vi "DOselector.vi"(8 "I/O element":T1(ring), 11 "value":bool) -> ()   [LabVIEW 2024]
uses:
  <vilib>/eio/EIONode/EIONode.xnode
  <vilib>/rvi/eio/common/nirviEmuTemplateMethod_errors.vi
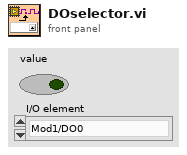
[diagram p1: front panel]
types:
  T1 = enum16{"Mod1/DO0", "Mod1/DO1", "Mod1/DO2", "Mod1/DO3", "Mod1/DO4", "Mod1/DO5", "Mod1/DO6", "Mod1/DO7", "Mod2/DIO0", "Mod2/DIO1", "Mod2/DIO2", "Mod2/DIO3", "Mod2/DIO4", "Mod2/DIO5", "Mod2/DIO6", "Mod2/DIO7"}
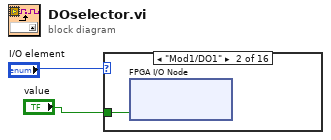
[diagram p0: block diagram]
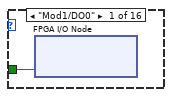
[diagram p2: hidden frame]
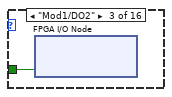
[diagram p3: hidden frame]
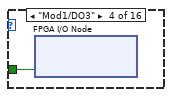
[diagram p4: hidden frame]
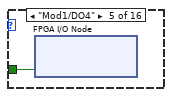
[diagram p5: hidden frame]
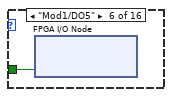
[diagram p6: hidden frame]
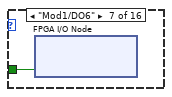
[diagram p7: hidden frame]
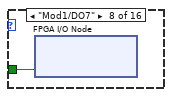
[diagram p8: hidden frame]
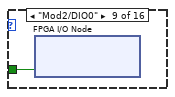
[diagram p9: hidden frame]
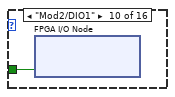
[diagram p10: hidden frame]
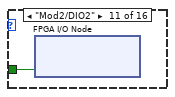
[diagram p11: hidden frame]
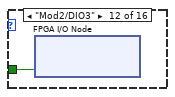
[diagram p12: hidden frame]
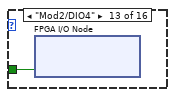
[diagram p13: hidden frame]
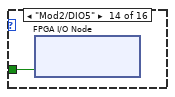
[diagram p14: hidden frame]
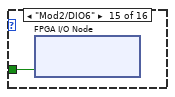
[diagram p15: hidden frame]
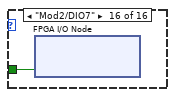
[diagram p16: hidden frame]
diagram:
  n1 = case shown="\"Mod1/DO1\"" "I/O element" {
    tunnel: "value" -> [w3 w4 w5 w6 w7 w8 w9 w10 w11 w12 w13 w14 w15 w16 w17 w18]
    frame "Mod1/DO0" {
      n2 = xnode "FPGA I/O Node"("Mod1/DO0"=w3) -> ()  [unwired: 2 in, 2 out]
    }
    frame "Mod1/DO1" {
      n3 = xnode "FPGA I/O Node"("Mod1/DO1"=w4) -> ()  [unwired: 2 in, 2 out]
    }
    frame "Mod1/DO2" {
      n4 = xnode "FPGA I/O Node"("Mod1/DO2"=w5) -> ()  [unwired: 2 in, 2 out]
    }
    frame "Mod1/DO3" {
      n5 = xnode "FPGA I/O Node"("Mod1/DO3"=w6) -> ()  [unwired: 2 in, 2 out]
    }
    frame "Mod1/DO4" {
      n6 = xnode "FPGA I/O Node"("Mod1/DO4"=w7) -> ()  [unwired: 2 in, 2 out]
    }
    frame "Mod1/DO5" {
      n7 = xnode "FPGA I/O Node"("Mod1/DO5"=w8) -> ()  [unwired: 2 in, 2 out]
    }
    frame "Mod1/DO6" {
      n8 = xnode "FPGA I/O Node"("Mod1/DO6"=w9) -> ()  [unwired: 2 in, 2 out]
    }
    frame "Mod1/DO7" {
      n9 = xnode "FPGA I/O Node"("Mod1/DO7"=w10) -> ()  [unwired: 2 in, 2 out]
    }
    frame "Mod2/DIO0" {
      n10 = xnode "FPGA I/O Node"("Mod2/DIO0"=w11) -> ()  [unwired: 2 in, 2 out]
    }
    frame "Mod2/DIO1" {
      n11 = xnode "FPGA I/O Node"("Mod2/DIO1"=w12) -> ()  [unwired: 2 in, 2 out]
    }
    frame "Mod2/DIO2" {
      n12 = xnode "FPGA I/O Node"("Mod2/DIO2"=w13) -> ()  [unwired: 2 in, 2 out]
    }
    frame "Mod2/DIO3" {
      n13 = xnode "FPGA I/O Node"("Mod2/DIO3"=w14) -> ()  [unwired: 2 in, 2 out]
    }
    frame "Mod2/DIO4" {
      n14 = xnode "FPGA I/O Node"("Mod2/DIO4"=w15) -> ()  [unwired: 2 in, 2 out]
    }
    frame "Mod2/DIO5" {
      n15 = xnode "FPGA I/O Node"("Mod2/DIO5"=w16) -> ()  [unwired: 2 in, 2 out]
    }
    frame "Mod2/DIO6" {
      n16 = xnode "FPGA I/O Node"("Mod2/DIO6"=w17) -> ()  [unwired: 2 in, 2 out]
    }
    frame "Mod2/DIO7" {
      n17 = xnode "FPGA I/O Node"("Mod2/DIO7"=w18) -> ()  [unwired: 2 in, 2 out]
    }
  }
